vi "两板卡同步_主卡采样时基同步_主卡外部触发.vi"() -> ()   [LabVIEW 2013]
doc: "This example demonstrates how to acquire a continuous data."
uses:
  <userlib>/ArtDAQ/_SubVI/ArtDAQ_CreateAIVoltageIEPEChan.vi
  <userlib>/ArtDAQ/_SubVI/ArtDAQ_CfgSampClkTiming.vi
  <userlib>/ArtDAQ/_SubVI/ArtDAQ_CfgDigEdgeStartTrig.vi
  <userlib>/ArtDAQ/_SubVI/ArtDAQ_Read Analog DBL NChan NSamp.vi
panel:
  in  "从卡触发接入端":string="RTSI1"
  in  "主卡触发导出端":string="RTSI1"
  in  "从卡采样时基接入端":string="RTSI8"
  in  "主卡采样时基导出端":string="RTSI8"
  in  "从卡物理通道":string(combo)="Dev1/ai0"
  out "从卡波形图":dbl[][](graph)
  in  "停止":bool
  out "主卡波形图":dbl[][](graph)
  in  "采样速率":dbl=10000.0 format="%#_13g"
  in  "主卡物理通道":string(combo)="Dev1/ai0"
  out "错误":errorcluster
  # "通道属性"
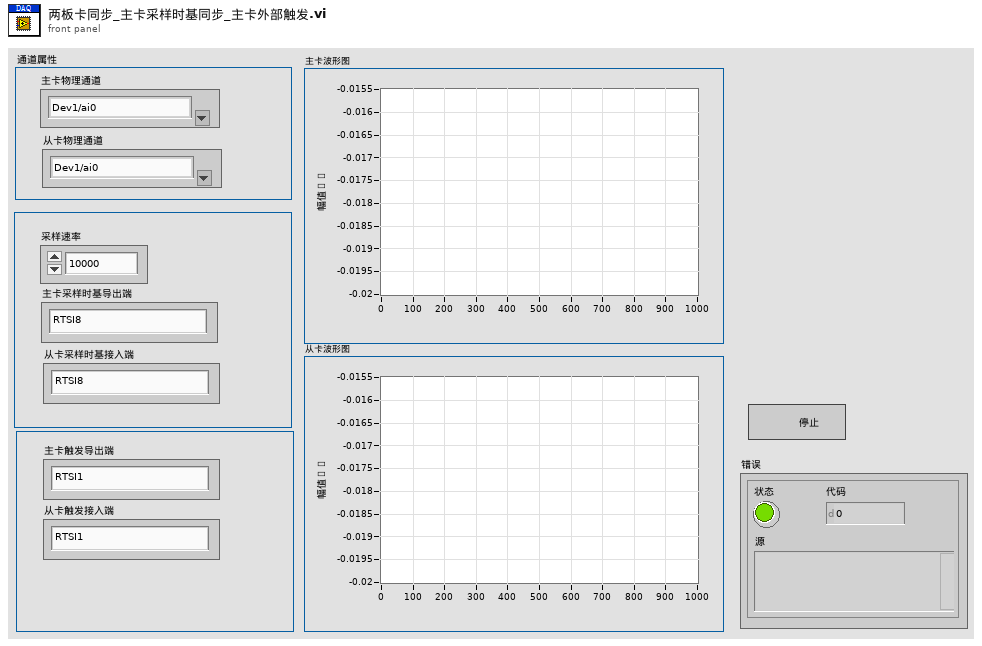
[diagram p1: front panel]
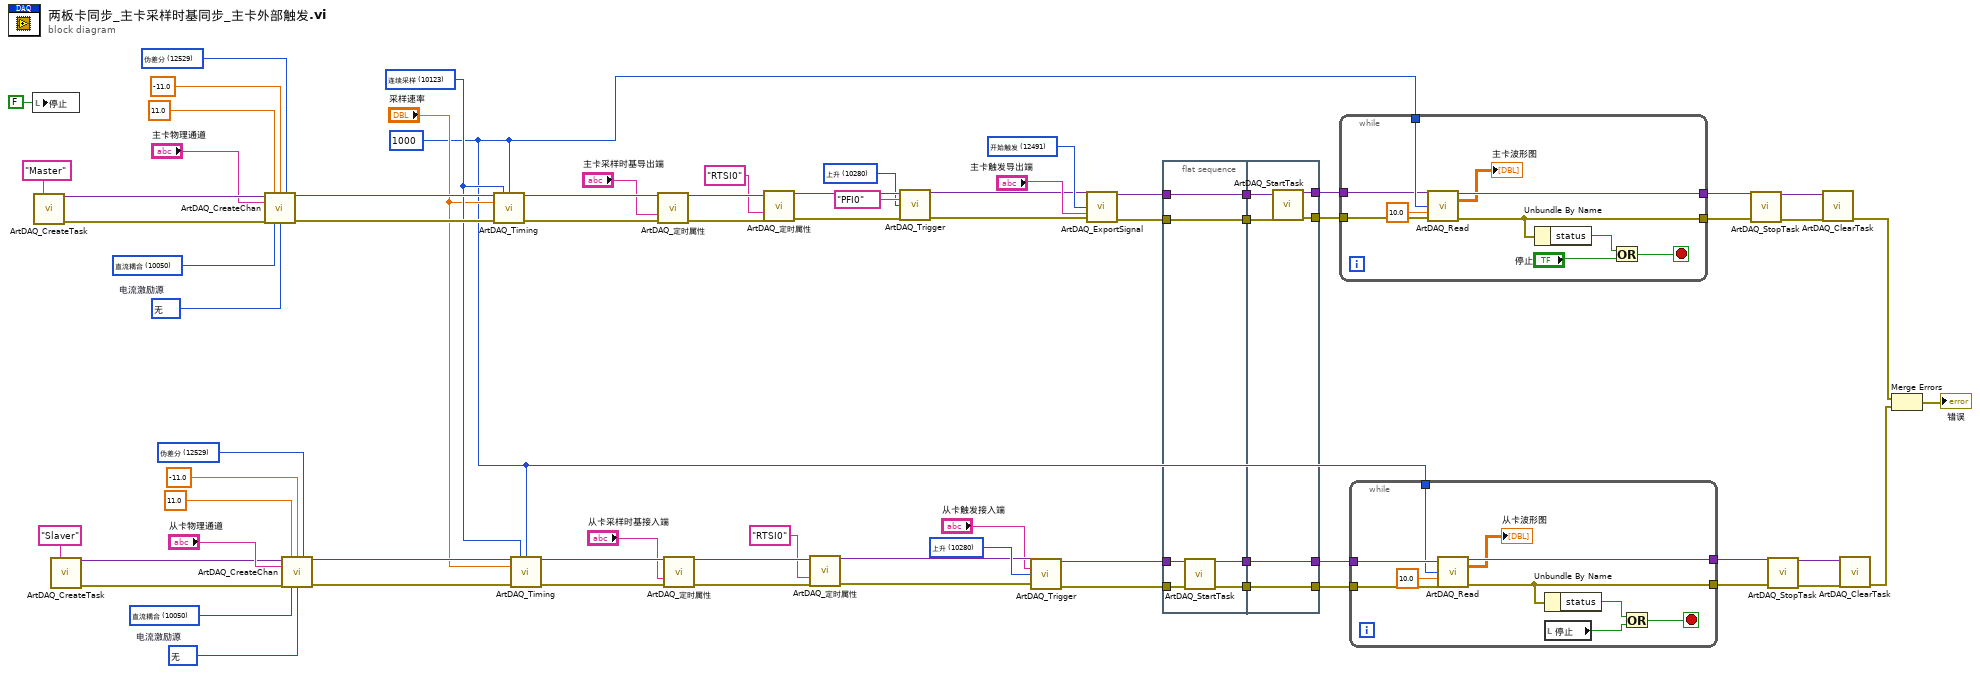
[diagram p0: block diagram]
diagram:
  w1 = 10280 items=["上升"=10280, "下降"=10171] ("边沿")
  w36 = 10280 items=["上升"=10280, "下降"=10171] ("斜率 2")
  w19 = 12491 items=["AI转换时钟"=12484, "10MHz参考时钟"=12536, "20MHz时基时钟"=12486, "采样时钟"=12487, "前移触发"=12488, "参考触发"=12490, "开始触发"=12491] ("信号")
  w37 = 1000 ("每通道采样数 2")
  w56 = 10050 items=["交流耦合"=10045, "直流耦合"=10050, "接地"=10066] ("耦合 2")
  w61 = 10050 items=["交流耦合"=10045, "直流耦合"=10050, "接地"=10066] ("耦合")
  w43 = 12529 items=["默认"=-1, "单端"=10083, "非参考单端"=10078, "差分"=10106, "伪差分"=12529] ("接线端配置 2")
  w70 = 12529 items=["默认"=-1, "单端"=10083, "非参考单端"=10078, "差分"=10106, "伪差分"=12529] ("接线端配置")
  w57 = 10230 items=["内部"=10200, "外部"=10167, "无"=10230]  # 电流激励源
  w39 = 10123 items=["有限点采样"=10178, "连续采样"=10123] ("SampleMode")
  w60 = 10230 items=["内部"=10200, "外部"=10167, "无"=10230]  # 电流激励源
  n1 = local write "停止"(FALSE ("停止")) -> ()
  n2 = call <userlib>:"ArtDAQ_CreateTask.vi"("任务名称"="Master") -> ("任务句柄"=w68:variant, "错误输出"=w73:errorcluster)  [unwired: 13 in]
  n3 = call <userlib>:"ArtDAQ_CreateTask.vi"("任务名称"="Slaver") -> ("任务句柄"=w47:variant, "错误输出"=w40:errorcluster)  [unwired: 13 in]
  n4 = call-poly <userlib>:"ArtDAQ_CreateChan.vi"("任务句柄"=w68, "最大值"=11.0 ("最大值(V)"), "最小值"=-11.0 ("最小值(V)"), "接线端配置"=w70, "物理通道"="主卡物理通道", "错误输入"=w73, "耦合方式"=w61, "电流激励源"=w60) -> ("任务句柄"=w62:variant, "错误输出"=w69:errorcluster)  [unwired: 6 in]
  n5 = call-poly <userlib>:"ArtDAQ_CreateChan.vi"("任务句柄"=w47, "最大值"=11.0 ("最大值(V) 2"), "最小值"=-11.0 ("最小值(V) 2"), "接线端配置"=w43, "物理通道"="从卡物理通道", "错误输入"=w40, "耦合方式"=w56, "电流激励源"=w57) -> ("任务句柄"=w55:variant, "错误输出"=w44:errorcluster)  [unwired: 6 in]
  n6 = call-poly <userlib>:"ArtDAQ_Timing.vi"("任务句柄"=w62, "采样模式"=w39, "每通道采样数"=w37, "采样率"="采样速率", "错误输入"=w69) -> ("任务句柄"=w32:variant, "错误输出"=w31:errorcluster)  [unwired: 9 in]
  n7 = call-poly <userlib>:"ArtDAQ_Timing.vi"("任务句柄"=w55, "采样模式"=w39, "每通道采样数"=w37, "采样率"="采样速率", "错误输入"=w44) -> ("任务句柄"=w30:variant, "错误输出"=w29:errorcluster)  [unwired: 9 in]
  n8 = call-poly "ArtDAQ_定时属性.vi"("任务句柄"=w32, "采样时基导出端"="主卡采样时基导出端", "错误输入"=w31) -> ("任务句柄"=w26:variant, "错误输出"=w27:errorcluster)  [unwired: 11 in]
  n9 = call-poly "ArtDAQ_定时属性.vi"("任务句柄"=w30, "采样时钟源"="从卡采样时基接入端", "错误输入"=w29) -> ("任务句柄"=w24:variant, "错误输出"=w23:errorcluster)  [unwired: 11 in]
  n10 = call-poly "ArtDAQ_定时属性.vi"("任务句柄"=w26, "同步脉冲源"="RTSI0", "错误输入"=w27) -> ("任务句柄"=w4:variant, "错误输出"=w6:errorcluster)  [unwired: 11 in]
  n11 = call-poly "ArtDAQ_定时属性.vi"("任务句柄"=w24, "同步脉冲源"="RTSI0", "错误输入"=w23) -> ("任务句柄"=w21:variant, "错误输出"=w22:errorcluster)  [unwired: 11 in]
  n12 = call-poly <userlib>:"ArtDAQ_Trigger.vi"("任务句柄"=w4, "触发源"="PFI0", "边沿"=w1, "错误输入"=w6) -> ("任务句柄"=w3:variant, "错误输出"=w5:errorcluster)  [unwired: 10 in]
  n13 = call-poly <userlib>:"ArtDAQ_Trigger.vi"("任务句柄"=w21, "触发源"="从卡触发接入端", "边沿"=w36, "错误输入"=w22) -> ("任务句柄"=w52:variant, "错误输出"=w53:errorcluster)  [unwired: 10 in]
  n14 = call <userlib>:"ArtDAQ_ExportSignal.vi"("任务句柄"=w3, "信号"=w19, "输出接线端"="主卡触发导出端", "错误输入"=w5) -> ("任务句柄"=w16:variant, "错误输出"=w14:errorcluster)  [unwired: 10 in]
  n15 = flat-sequence {
    tunnel: w53 -> [w79]
    tunnel: w52 -> [w78]
    tunnel: [w77] -> w18
    tunnel: [w76] -> w17
    tunnel: w16 -> [w75]
    tunnel: [w75] -> w15
    tunnel: w14 -> [w74]
    tunnel: [w74] -> w13
    tunnel: [w84] -> w45
    tunnel: [w85] -> w46
    tunnel: w18 -> [w85]
    tunnel: w17 -> [w84]
    tunnel: w15 -> [w83]
    tunnel: w13 -> [w82]
    tunnel: [w81] -> w12
    tunnel: [w80] -> w11
    frame #0 {
      n16 = call <userlib>:"ArtDAQ_StartTask.vi"("任务句柄"=w78, "错误输入"=w79) -> ("任务句柄"=w76:variant, "错误输出"=w77:errorcluster)  [unwired: 12 in]
    }
    frame #1 {
      n17 = call <userlib>:"ArtDAQ_StartTask.vi"("任务句柄"=w83, "错误输入"=w82) -> ("任务句柄"=w81:variant, "错误输出"=w80:errorcluster)  [unwired: 12 in]
    }
  }
  n18 = while {
    tunnel: w37 -> [w95]
    tunnel: [w93] -> w67
    tunnel: [w92] -> w66
    tunnel: w12 -> [w87]
    tunnel: w11 -> [w86]
    stop <- w90 stop-if-true
    n19 = call-poly <userlib>:"ArtDAQ_Read.vi"("任务句柄"=w87, "每通道采样数"=w95, "超时s"=10.0 ("Timeout"), "错误输入"=w86) -> ("任务句柄"=w93:variant, "数据"=→"主卡波形图":dbl[][], "错误输出"=w92:errorcluster)  [unwired: 8 in, 1 out]
    n20 = Unbundle By Name(w92) -> ("status"=w91:bool)
    n21 = Or(x=w91, y="停止") -> (x .or. y?=w90:bool)
  }
  n22 = while {
    tunnel: w45 -> [w105]
    tunnel: w46 -> [w104]
    tunnel: w37 -> [w103]
    tunnel: [w101] -> w48
    tunnel: [w100] -> w49
    stop <- w97 stop-if-true
    n23 = call-poly <userlib>:"ArtDAQ_Read.vi"("任务句柄"=w105, "每通道采样数"=w103, "超时s"=10.0 ("Timeout"), "错误输入"=w104) -> ("任务句柄"=w101:variant, "数据"=→"从卡波形图":dbl[][], "错误输出"=w100:errorcluster)  [unwired: 8 in, 1 out]
    n24 = Unbundle By Name(w100) -> ("status"=w99:bool)
    n25 = local read "停止"() -> (w96:bool)
    n26 = Or(x=w99, y=w96) -> (x .or. y?=w97:bool)
  }
  n27 = call <userlib>:"ArtDAQ_StopTask.vi"("任务句柄"=w67, "错误输入"=w66) -> ("任务句柄"=w65:variant, "错误输出"=w64:errorcluster)  [unwired: 12 in]
  n28 = call <userlib>:"ArtDAQ_StopTask.vi"("任务句柄"=w48, "错误输入"=w49) -> ("任务句柄"=w50:variant, "错误输出"=w51:errorcluster)  [unwired: 12 in]
  n29 = call <userlib>:"ArtDAQ_ClearTask.vi"("任务句柄"=w65, "错误输入"=w64) -> ("错误输出"=w35:errorcluster)  [unwired: 13 in]
  n30 = call <userlib>:"ArtDAQ_ClearTask.vi"("任务句柄"=w50, "错误输入"=w51) -> ("错误输出"=w34:errorcluster)  [unwired: 13 in]
  n31 = Merge Errors(w35, w34) -> (→"错误":errorcluster)
